vi "设备配置界面.vi"() -> ()   [LabVIEW 2016, in "环境动力监测库.lvlib"]
panel:
  in  "配置说明":bool
  in  "设置默认配置":bool
  in  "一键恢复默认设置":bool
  in  "add2":bool
  in  "串口连接":T1(ring)
  in  "设备列表":i32(listbox)=-1
  in  "add":bool
  in  "IO连接":T2(ring)
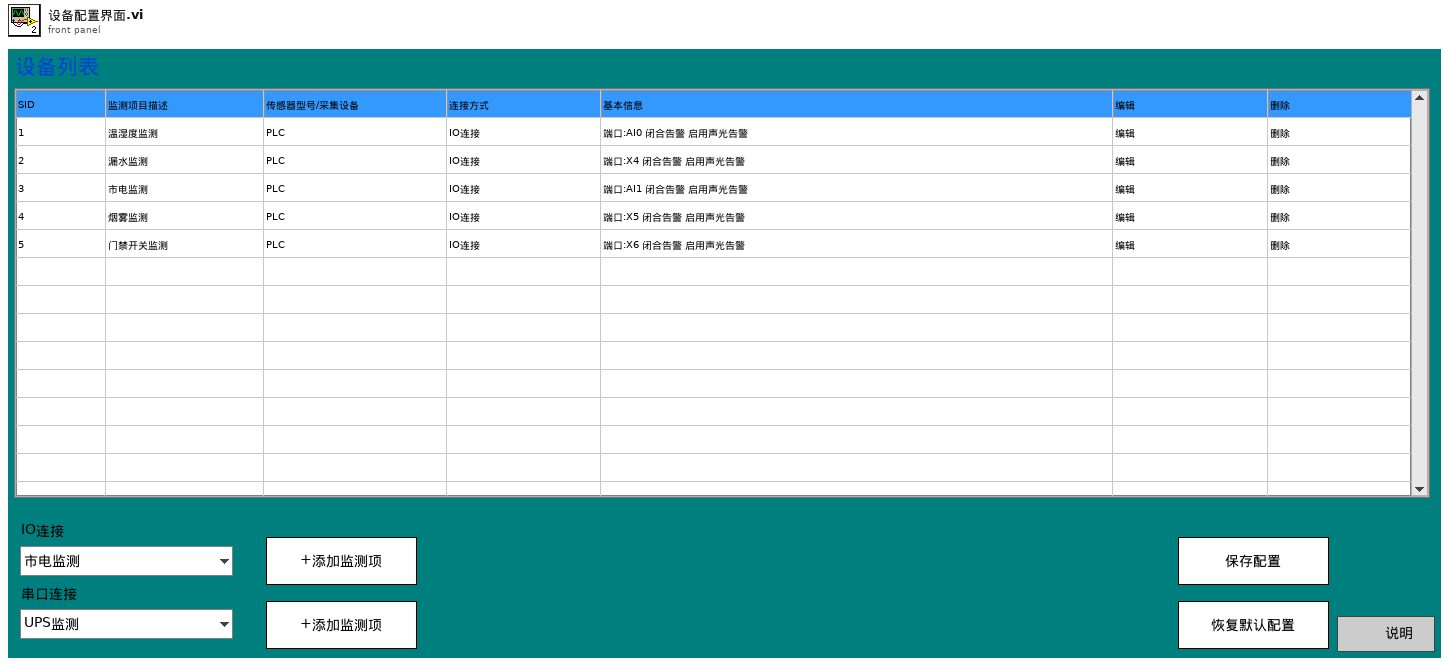
[diagram p1: front panel]
types:
  T1 = enum16{"UPS监测", "空调监测", "蓄电池监测", "GPS监测", "北斗监测", "智能门禁监测"}
  T2 = enum16{"市电监测", "用水量监测", "烟雾监测", "温湿度监测", "振动监测", "红外入侵监测", "漏水监测", "门禁开关监测", "视频监测", "冰箱监测", "排气扇监测", "废液监测"}
  T3 = cluster{"监测项描述:输出":string, "端口":enum16{"AI0", "AI1", "AI2", "AI3", "AI4", "DI0", "DI1", "DI2", "DI3", "DI4", "DI5", "DI6", "DI7", "DO0", "DO1", "DO2", "DO3", "DO4", "DO5", "DO6", "DO7", "X0", "X1", "X2", "X3", "X4", "X5", "X6", "X7", "X8", "X9", "X10", "X11", "X12", "X13", "X14", "X15", "X16", "X17", "X18", "X19", "X20", "X21", "X22", "X23", "Y0", "Y1", "Y2", "Y3", "Y4", "Y5", "Y6", "Y7", "Y8", "Y9", "Y10", "Y11", "Y12", "Y13", "Y14", "Y15", "Y16", "Y17", "Y18", "Y19", "Y20", "Y21", "Y22", "Y23", "Y24", "Y25", "Y26", "Y27", "Y28", "Y29", "Y30", "Y31", "Y32", "Y33", "Y34", "Y35", "Y36", "Y37", "Y38", "Y39"}, "告警方式":enum32{"禁用告警", "闭合告警", "断开告警"}, "传感器型号":enum16{"PLC", "ZLAN", "ART"}, "声光告警启用":bool}
  T4 = cluster{"监测项描述:输出":string, "连接方式":enum16{"串口", "TCP"}, "端口":string, "IP address:":string, "Port:":string, "站号":u64, "传感器型号":string, "波特率":u64, "data bits":u64, "停止位":u16, "奇偶校验":u16, "声光告警启用":bool}
  T5 = typedef "LVPoint32TypeDef.ctl" = cluster{"Horizontal":i32, "Vertical":i32}
  T6 = typedef "LVRowAndColumnTypeDef.ctl" = cluster{"Row":i32, "Column":i32}
  T7 = enum16{"Left Button", "Center Button", "Right Button", "Window Close"}
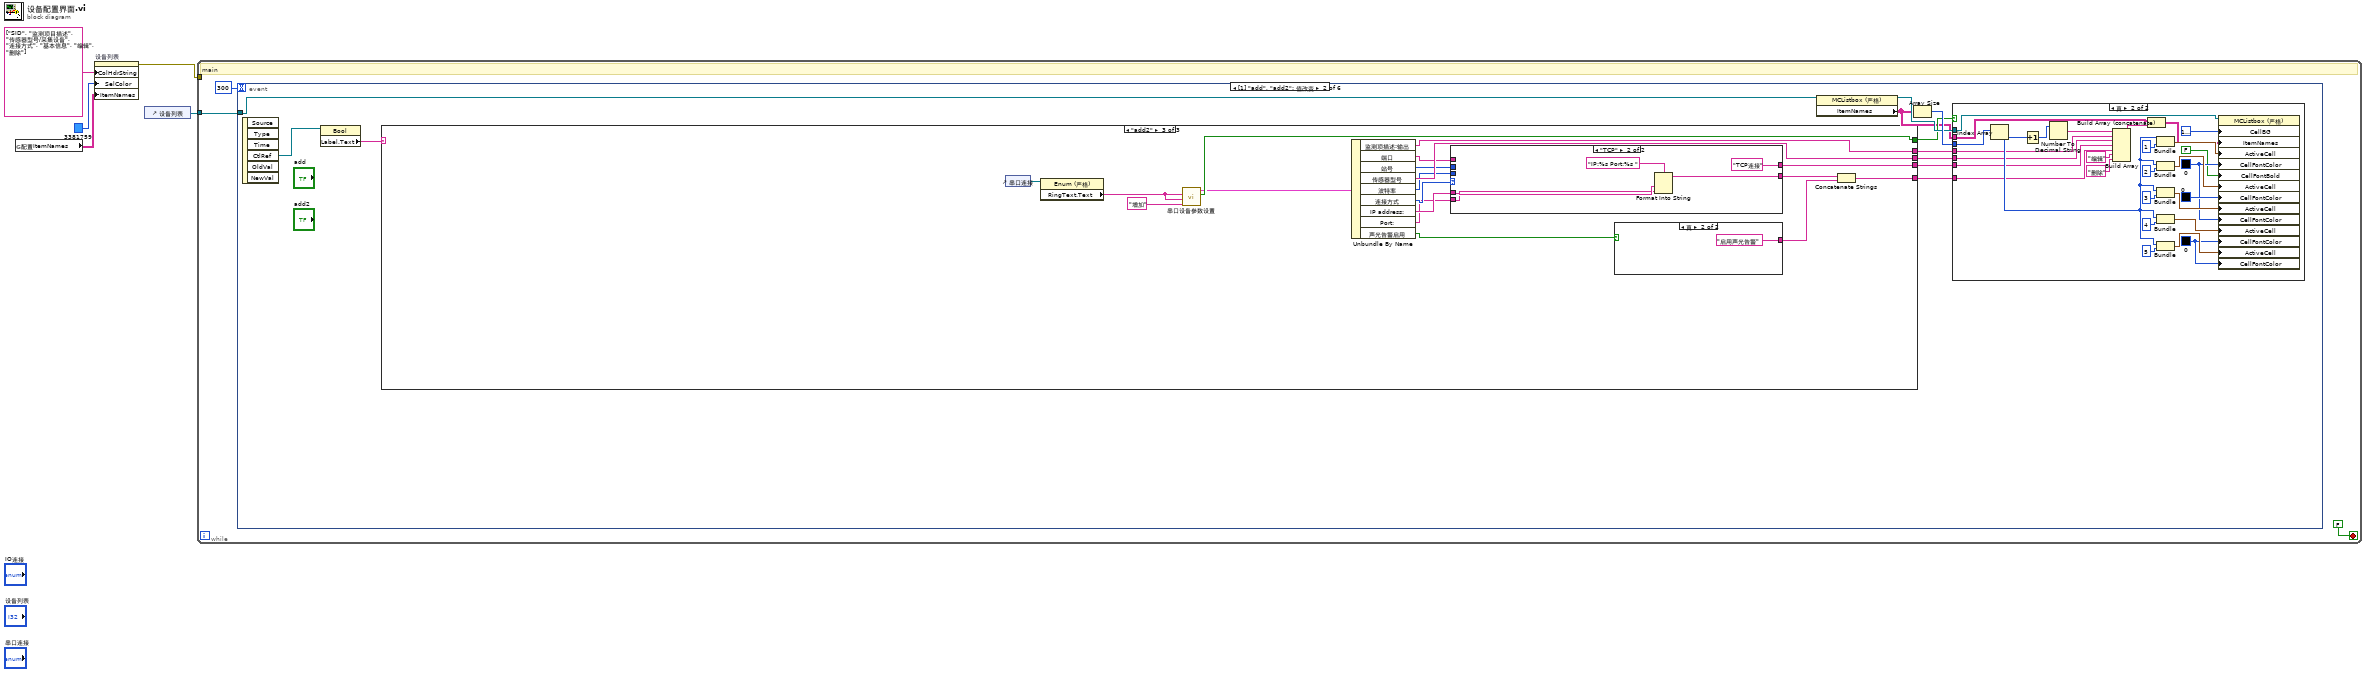
[diagram p0: block diagram]
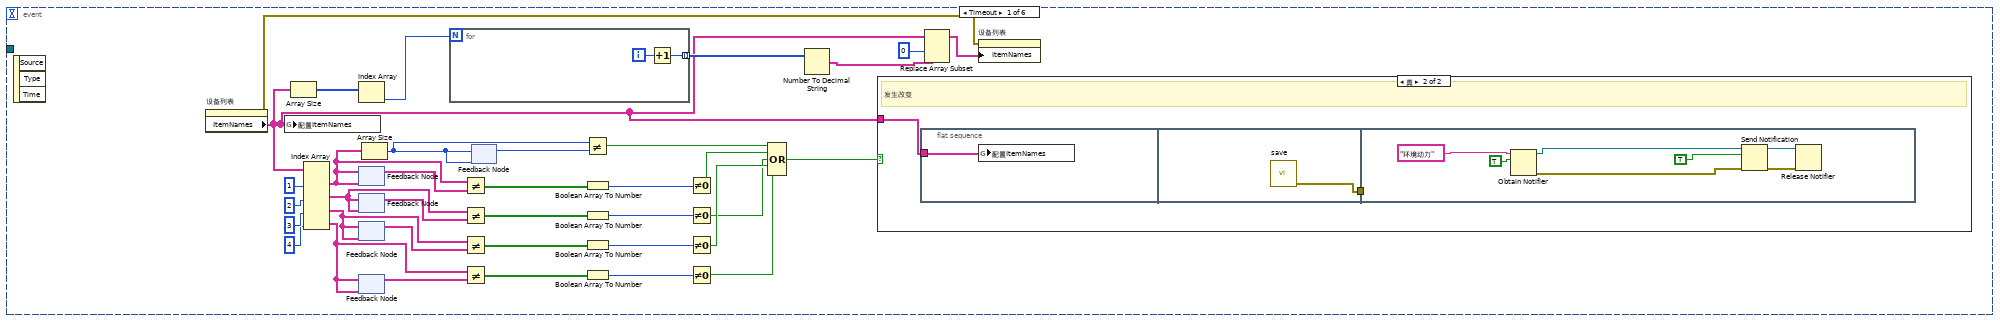
[diagram p2: hidden frame]
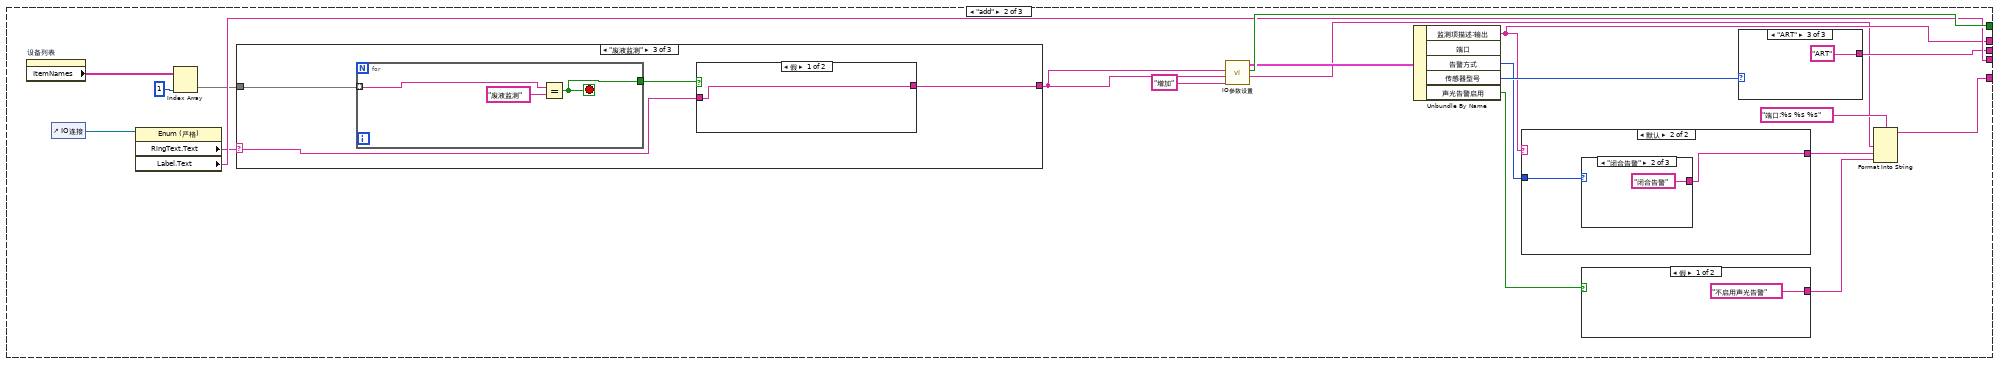
[diagram p5: hidden frame]
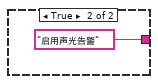
[diagram p6: hidden frame]
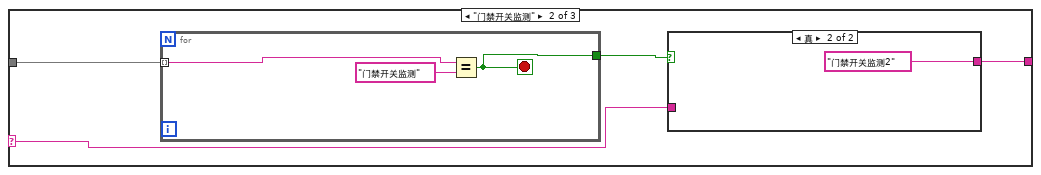
[diagram p8: hidden frame]
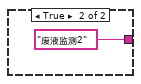
[diagram p10: hidden frame]
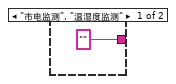
[diagram p11: hidden frame]
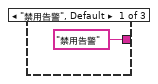
[diagram p12: hidden frame]
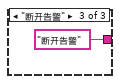
[diagram p13: hidden frame]
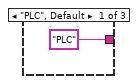
[diagram p14: hidden frame]
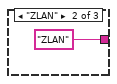
[diagram p15: hidden frame]
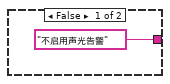
[diagram p16: hidden frame]
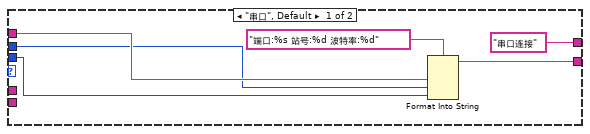
[diagram p17: hidden frame]
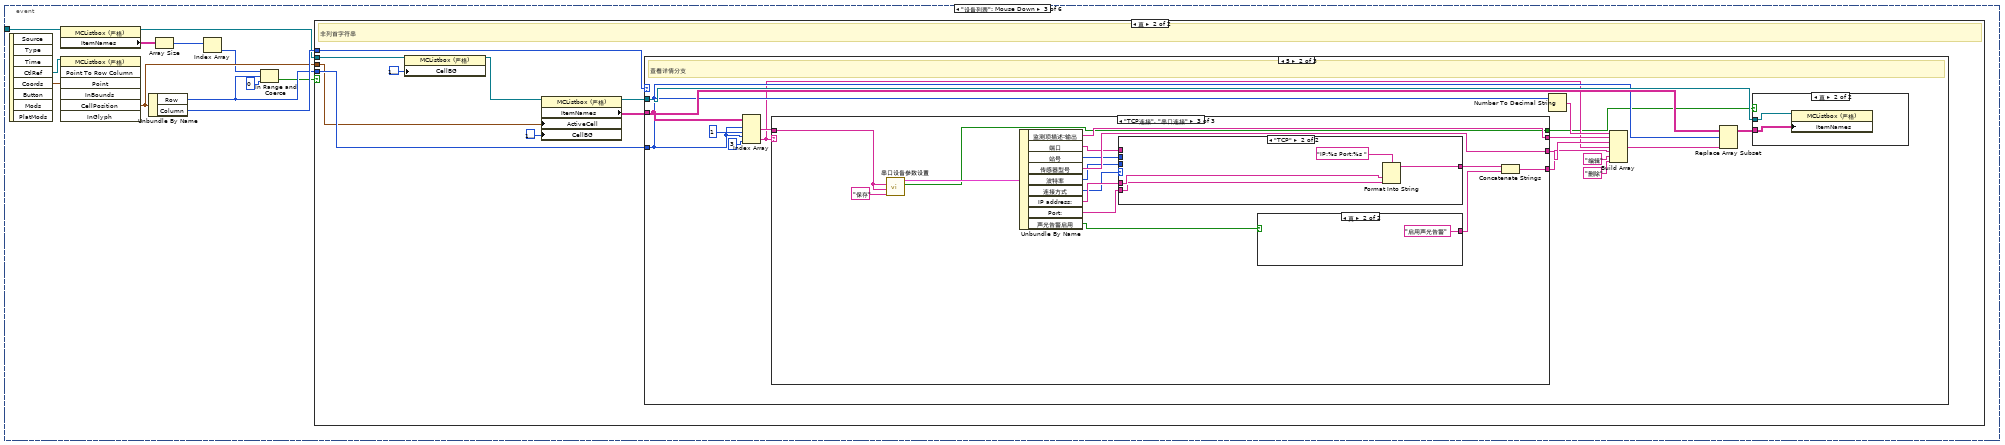
[diagram p19: hidden frame]
diagram:
  n1 = global read "断电保存全局变量.vi" "配置ItemNames"() -> (w1:string[][])
  n2 = property on="设备列表" class="MCListbox (严格)"("ColHdrString"=string[] ["SID", "监测项目描述", "传感器型号/采集设备", "连接方式", "基本信息", "编辑", "删除"] ("列首字符串[]"), "SelColor"=u32 3381759, "ItemNames"=w1) -> (error out=w4:errorcluster)  [unwired: 2 in, 1 out]
  n3 = control-ref of="设备列表"() -> (w5:refnum<vi>)
  n4 = while {
    tunnel: w5 -> [w7]
    tunnel: w4 -> [_]
    stop <- FALSE stop-if-true
    # "main"
    n5 = event shown="[1] \"add\", \"add2\": 值改变" {
      selector: _ -> [_ _ _ _ _ _]
      dyn-events: _ -> [_ _ _ _ _ _]
      timeout: 300 -> [_ _ _ _ _ _]
      tunnel: w7 -> [_ w68 w184 _ _ _]
      event Timeout {
        n6 = event-data() -> ()  [unwired: 1 in, 3 out]
        n7 = property on="设备列表" class="MCListbox (严格)"() -> (error out=w43:errorcluster, "ItemNames"=w9:string[][])  [unwired: 2 in, 1 out]
        n8 = global write "断电保存全局变量.vi" "配置ItemNames"(w9) -> ()
        n9 = Array Size(array=w9) -> (size(s)=w44:i32[])
        n10 = Index Array(array=w9, index (col) #1=1 ("禁用的索引 (列)"), index (col) #2=2 ("索引 (列)"), index (col) #3=3 ("索引 (列)"), index (col) #4=4 ("索引 (列)")) -> (element #1=w14:string[], element #2=w21:string[], element #3=w20:string[], element #4=w19:string[])  [unwired: 4 in]
        n11 = Index Array(array=w44) -> (element=w38:i32)  [unwired: 1 in]
        n12 = feedback-in #1(w14) -> ()
        n13 = feedback #1(w14) -> (w33:string[])
        n14 = feedback #2(w21) -> (w28:string[])
        n15 = feedback-in #2(w21) -> ()
        n16 = feedback #3(w20) -> (w27:string[])
        n17 = feedback-in #3(w20) -> ()
        n18 = feedback #4(w19) -> (w22:string[])
        n19 = feedback-in #4(w19) -> ()
        n20 = Array Size(array=w14) -> (size(s)=w12:i32)
        n21 = for {
          N: w38 -> [_]
          tunnel: [w56] -> w42 mode=indexing
          i -> [w57]
          n22 = Increment(x=w57) -> (x+1=w56:i32)
        }
        n23 = Not Equal?(x=w14, y=w33) -> (x != y?=w13:bool[])
        n24 = Not Equal?(x=w21, y=w28) -> (x != y?=w29:bool[])
        n25 = Not Equal?(x=w20, y=w27) -> (x != y?=w26:bool[])
        n26 = Not Equal?(x=w19, y=w22) -> (x != y?=w23:bool[])
        n27 = feedback #5(w12) -> (w11:i32)
        n28 = feedback-in #5(w12) -> ()
        n29 = Not Equal?(x=w12, y=w11) -> (x != y?=w10:bool)
        n30 = Boolean Array To Number(Boolean array=w13) -> (number=w32:u32)
        n31 = Boolean Array To Number(Boolean array=w29) -> (number=w30:u32)
        n32 = Boolean Array To Number(Boolean array=w26) -> (number=w25:u32)
        n33 = Boolean Array To Number(Boolean array=w23) -> (number=w24:u32)
        n34 = Not Equal To 0?(x=w32) -> (x != 0?=w31:bool)
        n35 = Not Equal To 0?(x=w30) -> (x != 0?=w16:bool)
        n36 = Not Equal To 0?(x=w25) -> (x != 0?=w17:bool)
        n37 = Not Equal To 0?(x=w24) -> (x != 0?=w18:bool)
        n38 = Compound Arithmetic op=OR ("复合运算")(w10, w31, w16, w17, w18) -> (w15:bool)
        n39 = Number To Decimal String(number=w42) -> (decimal integer string=w41:string[])  [unwired: 1 in]
        n40 = case shown="真" w15 {
          tunnel: w9 -> [_ w46]
          frame False {
          }
          frame True {
            # "发生改变"
            n41 = flat-sequence {
              tunnel: w46 -> [w47]
              tunnel: [w48] -> w45
              tunnel: w45 -> [_]
              frame #0 {
                n42 = global write "断电保存全局变量.vi" "配置ItemNames"(w47) -> ()
              }
              frame #1 {
                n43 = call "save.vi"() -> ("error out"=w48:errorcluster)  [unwired: 11 in]
              }
              frame #2 {
                n44 = Obtain Notifier(name (unnamed)="环境动力" ("名称（未命名）"), notification data type=TRUE) -> (notifier out=w51:refnum<notifier>, error out=w52:errorcluster)  [unwired: 2 in, 1 out]
                n45 = Send Notification(notification=TRUE ("通知"), notifier=w51, error in (no error)=w52) -> (notifier out=w54:refnum<notifier>, error out=w55:errorcluster)
                n46 = Release Notifier(notifier=w54, error in (no error)=w55) -> ()  [unwired: 1 in, 3 out]
              }
            }
          }
        }
        n47 = Replace Array Subset(array=w9, new element=w41, index (col)=0 ("禁用的索引 (列)")) -> (w39:string[][])  [unwired: 1 in]
        n48 = property on="设备列表" class="MCListbox (严格)"(error in=w43, "ItemNames"=w39) -> ()  [unwired: 1 in, 2 out]
      }
      event "add", "add2": Value Change {
        n49 = event-data() -> ("CtlRef"=w63:refnum<vi>)  [unwired: 1 in, 5 out]
        n50 = property class="Bool"(reference=w63) -> ("Label.Text"=w62:string)  [unwired: 1 in, 2 out]
        n51 = case shown="\"add2\"" w62 {
          tunnel: [_ w88 w135] -> w65
          tunnel: [_ w85 w119] -> w61
          tunnel: [_ w77 w131] -> w60
          tunnel: [_ w80 w130] -> w59
          tunnel: [_ w82 w120] -> w58
          frame "假", Default {
          }
          frame "add" {
            n52 = property on="设备列表" class="MCListbox (严格)"() -> ("ItemNames"=w71:string[][])  [unwired: 2 in, 2 out]
            n53 = control-ref of="IO连接"() -> (w86:refnum<vi>)
            n54 = property class="Enum (严格)"(reference=w86) -> ("RingText.Text"=w73:string, "Label.Text"=w85:string)  [unwired: 1 in, 2 out]
            n55 = Index Array(array=w71, index (col)=1 ("禁用的索引 (列)")) -> (element=w70:string[])  [unwired: 1 in]
            n56 = case shown="\"废液监测\"" w73 {
              selector: w73 -> [w91 w92 w101]
              tunnel: [w91 w95 w104] -> w76
              tunnel: w70 -> [_ w93 w102]
              frame "假", Default {
              }
              frame "门禁开关监测" {
                n57 = for {
                  tunnel: w93 -> [w100] mode=indexing
                  tunnel: [w98] -> w94
                  stop <- w98 stop-if-true
                  n58 = Equal?(x=w100, y="门禁开关监测") -> (x = y?=w98:bool)
                }
                n59 = case shown="真" w94 {
                  tunnel: w92 -> [w96 _]
                  tunnel: [w96 "门禁开关监测2" ("y")] -> w95
                  frame False {
                  }
                  frame True {
                  }
                }
              }
              frame "废液监测" {
                n60 = for {
                  tunnel: w102 -> [w109] mode=indexing
                  tunnel: [w107] -> w103
                  stop <- w107 stop-if-true
                  n61 = Equal?(x=w109, y="废液监测") -> (x = y?=w107:bool)
                }
                n62 = case shown="假" w103 {
                  tunnel: w101 -> [w105 _]
                  tunnel: [w105 "废液监测2" ("y")] -> w104
                  frame False {
                  }
                  frame True {
                  }
                }
              }
            }
            n63 = call "IO参数设置.vi"("布尔文本.文本"="增加", "section (optional)"=w76, "监测项描述"=w76) -> ("端口"=w69:string, "增加？"=w88:bool, "簇1输出"=w84:T3)  [unwired: 6 in]
            n64 = Unbundle By Name(w84) -> ("监测项描述:输出"=w77:string, "告警方式"=w79:enum32{"禁用告警", "闭合告警", "断开告警"}, "传感器型号"=w81:enum16{"PLC", "ZLAN", "ART"}, "声光告警启用"=w75:bool)  [unwired: 1 out]
            n65 = case shown="默认" w77 {
              tunnel: w79 -> [_ w112]
              tunnel: ["" w111] -> w78
              frame "市电监测", "温湿度监测" {
              }
              frame Default {
                n66 = case shown="\"闭合告警\"" w112 {
                  tunnel: ["禁用告警" "闭合告警" "断开告警"] -> w111
                  frame "禁用告警", Default {
                  }
                  frame "闭合告警" {
                  }
                  frame "断开告警" {
                  }
                }
              }
            }
            n67 = case shown="假" w75 {
              tunnel: ["不启用声光告警" "启用声光告警"] -> w74
              frame False {
              }
              frame True {
              }
            }
            n68 = case shown="\"ART\"" w81 {
              tunnel: ["PLC" "ZLAN" "ART"] -> w80
              frame "PLC", Default {
              }
              frame "ZLAN" {
              }
              frame "ART" {
              }
            }
            n69 = Format Into String(format string="端口:%s %s %s" ("格式字符串"), w69, w78, w74) -> (resulting string=w82:string)  [unwired: 2 in, 1 out]
          }
          frame "add2" {
            n70 = control-ref of="串口连接"() -> (w133:refnum<vi>)
            n71 = property class="Enum (严格)"(reference=w133) -> ("RingText.Text"=w134:string)  [unwired: 1 in, 2 out]
            n72 = call "串口设备参数设置.vi"("布尔文本.文本"="增加" ("section (optional)"), "section (optional)"=w134, "监测项描述"=w134) -> ("布尔"=w135:bool, "输出簇"=w132:T4)  [unwired: 7 in]
            n73 = Unbundle By Name(w132) -> ("监测项描述:输出"=w131:string, "端口"=w128:string, "站号"=w127:u64, "传感器型号"=w130:string, "波特率"=w126:u64, "连接方式"=w129:enum16{"串口", "TCP"}, "IP address:"=w125:string, "Port:"=w124:string, "声光告警启用"=w123:bool)
            n74 = case shown="\"TCP\"" w129 {
              tunnel: [w143 w146] -> w121
              tunnel: w128 -> [w142 _]
              tunnel: w127 -> [w141 _]
              tunnel: w126 -> [w140 _]
              tunnel: w125 -> [_ w148]
              tunnel: w124 -> [_ w147]
              tunnel: ["串口连接" "TCP连接"] -> w119
              frame "串口", Default {
                n75 = Format Into String(format string="端口:%s 站号:%d 波特率:%d" ("格式字符串"), w142, w141, w140) -> (resulting string=w143:string)  [unwired: 2 in, 1 out]
              }
              frame "TCP" {
                n76 = Format Into String(format string="IP:%s Port:%s " ("格式字符串"), w148, w147) -> (resulting string=w146:string)  [unwired: 2 in, 1 out]
              }
            }
            n77 = case shown="真" w123 {
              tunnel: ["不启用声光告警" ("格式字符串") "启用声光告警" ("格式字符串")] -> w122
              frame False {
              }
              frame True {
              }
            }
            n78 = Concatenate Strings(w121, w122) -> (w120:string)
          }
        }
        n79 = property class="MCListbox (严格)"(reference=w68) -> (reference out=w66:refnum<vi>, "ItemNames"=w64:string[][])  [unwired: 1 in, 1 out]
        n80 = Array Size(array=w64) -> (size(s)=w67:i32[])
        n81 = case shown="真" w65 {
          tunnel: w64 -> [_ w177]
          tunnel: w67 -> [_ w176]
          tunnel: w66 -> [_ w174]
          tunnel: w61 -> [_ w156]
          tunnel: w60 -> [_ w153]
          tunnel: w59 -> [_ w152]
          tunnel: w58 -> [_ w151]
          frame False {
          }
          frame True {
            w157 = u32 0 ("颜色盒")
            w164 = u32 0 ("颜色盒")
            n82 = Index Array(array=w176) -> (element=w159:i32)  [unwired: 1 in]
            n83 = Increment(x=w159) -> (x+1=w175:i32)
            n84 = Number To Decimal String(number=w175) -> (decimal integer string=w154:string)  [unwired: 1 in]
            n85 = Build Array(w154, w153, w152, w156, w151, "编辑" ("元素"), "删除" ("元素")) -> (w178:string[])
            n86 = Build Array (concatenate)(w177, w178) -> (w155:string[][])
            n87 = Bundle(w159, "Column"=1) -> (w165:cluster{i32, "Column":i32})  [unwired: 1 in]
            n88 = Bundle(w159, "Column"=2) -> (w171:cluster{i32, "Column":i32})  [unwired: 1 in]
            n89 = Bundle(w159, "Column"=3) -> (w168:cluster{i32, "Column":i32})  [unwired: 1 in]
            n90 = Bundle(w159, "Column"=4) -> (w166:cluster{i32, "Column":i32})  [unwired: 1 in]
            n91 = Bundle(w159, "Column"=5) -> (w158:cluster{i32, "Column":i32})  [unwired: 1 in]
            n92 = property class="MCListbox (严格)"(reference=w174, "CellBG"=u32 16777216 ("颜色盒"), "ItemNames"=w155, "ActiveCell"=w165, "CellFontColor"=w164, "CellFontBold"=FALSE ("活动单元格:单元格字体:斜体"), "ActiveCell"=w171, "CellFontColor"=u32 0 ("颜色盒"), "ActiveCell"=w168, "CellFontColor"=w164, "ActiveCell"=w166, "CellFontColor"=w157, "ActiveCell"=w158, "CellFontColor"=w157) -> ()  [unwired: 1 in, 2 out]
          }
        }
      }
      event "设备列表": Mouse Down {
        n93 = event-data() -> ("CtlRef"=w190:refnum<vi>, "Coords"=w188:T5)  [unwired: 1 in, 6 out]
        n94 = property class="MCListbox (严格)"(reference=w184) -> (reference out=w180:refnum<vi>, "ItemNames"=w183:string[][])  [unwired: 1 in, 1 out]
        n95 = invoke class="MCListbox (严格)" method="Point To Row Column"(reference=w190, "Point"=w188) -> ("CellPosition"=w187:T6)  [unwired: 5 in, 6 out]
        n96 = Unbundle By Name(w187) -> ("Row"=w186:i32, "Column"=w189:i32)
        n97 = Array Size(array=w183) -> (size(s)=w182:i32[])
        n98 = Index Array(array=w182) -> (element=w181:i32)  [unwired: 1 in]
        n99 = In Range and Coerce(upper limit=w181, x=w186, lower limit=0 ("下限")) -> (In Range?=w179:bool)  [unwired: 1 out]
        n100 = case shown="真" w179 {
          tunnel: w189 -> [_ w198]
          tunnel: w186 -> [_ w197]
          tunnel: w187 -> [_ w195]
          tunnel: w180 -> [_ w192]
          frame False {
          }
          frame True {
            # "非列首字符串"
            n101 = property class="MCListbox (严格)"(reference=w192, "CellBG"=u32 16777216) -> (reference out=w193:refnum<vi>)  [unwired: 1 in, 1 out]
            n102 = property class="MCListbox (严格)"(reference=w193, "ActiveCell"=w195, "CellBG"=u32 16777216) -> (reference out=w196:refnum<vi>, "ItemNames"=w199:string[][])  [unwired: 1 in, 1 out]
            n103 = case shown="5" w198 {
              tunnel: w199 -> [_ w211 w277]
              tunnel: w197 -> [_ w206 w275]
              tunnel: w196 -> [_ w212 w276]
              frame 0, Default {
              }
              frame 5 {
                # "查看详情分支"
                n104 = Index Array(array=w211, index (row) #1=w206, index (col) #1=1 ("禁用的索引 (列)"), index (row) #2=w206, index (col) #2=3 ("禁用的索引 (列)")) -> (element #1=w214:string, element #2=w201:string)
                n105 = case shown="\"TCP连接\", \"串口连接\"" w201 {
                  tunnel: w214 -> [_ w226 w253]
                  tunnel: [_ w222 w256] -> w204
                  tunnel: [_ w228 w244] -> w202
                  tunnel: [_ w224 w255] -> w203
                  tunnel: [_ w227 w254] -> w200
                  frame "假", Default {
                  }
                  frame "IO连接" {
                    n106 = call "IO参数设置.vi"("布尔文本.文本"="保存", "section (optional)"=w226, "监测项描述"=w226) -> ("端口"=w218:string, "增加？"=w227:bool, "簇1输出"=w229:T3)  [unwired: 6 in]
                    n107 = Unbundle By Name(w229) -> ("监测项描述:输出"=w222:string, "告警方式"=w223:enum32{"禁用告警", "闭合告警", "断开告警"}, "传感器型号"=w225:enum16{"PLC", "ZLAN", "ART"}, "声光告警启用"=w220:bool)  [unwired: 1 out]
                    n108 = case shown="\"市电监测\", \"温湿度监测\"" w222 {
                      tunnel: w223 -> [_ w236]
                      tunnel: ["" w235] -> w221
                      frame "市电监测", "温湿度监测" {
                      }
                      frame Default {
                        n109 = case shown="\"禁用告警\", 默认" w236 {
                          tunnel: ["禁用告警" "闭合告警" "断开告警"] -> w235
                          frame "禁用告警", Default {
                          }
                          frame "闭合告警" {
                          }
                          frame "断开告警" {
                          }
                        }
                      }
                    }
                    n110 = case shown="真" w220 {
                      tunnel: ["不启用声光告警" ("格式字符串") "启用声光告警" ("格式字符串")] -> w219
                      frame False {
                      }
                      frame True {
                      }
                    }
                    n111 = case shown="\"ART\"" w225 {
                      tunnel: ["PLC" "ZLAN" "ART"] -> w224
                      frame "PLC", Default {
                      }
                      frame "ZLAN" {
                      }
                      frame "ART" {
                      }
                    }
                    n112 = Format Into String(format string="端口:%s %s %s" ("格式字符串"), w218, w221, w219) -> (resulting string=w228:string)  [unwired: 2 in, 1 out]
                  }
                  frame "TCP连接", "串口连接" {
                    n113 = call "串口设备参数设置.vi"("布尔文本.文本"="保存", "section (optional)"=w253, "监测项描述"=w253) -> ("布尔"=w254:bool, "输出簇"=w257:T4)  [unwired: 7 in]
                    n114 = Unbundle By Name(w257) -> ("监测项描述:输出"=w256:string, "端口"=w249:string, "站号"=w248:u64, "传感器型号"=w255:string, "波特率"=w247:u64, "连接方式"=w250:enum16{"串口", "TCP"}, "IP address:"=w252:string, "Port:"=w251:string, "声光告警启用"=w246:bool)
                    n115 = case shown="\"TCP\"" w250 {
                      tunnel: [w264 w266] -> w245
                      tunnel: w249 -> [w263 _]
                      tunnel: w248 -> [w262 _]
                      tunnel: w247 -> [w261 _]
                      tunnel: w252 -> [_ w268]
                      tunnel: w251 -> [_ w267]
                      frame "串口", Default {
                        n116 = Format Into String(format string="端口:%s 站号:%d 波特率:%d" ("格式字符串"), w263, w262, w261) -> (resulting string=w264:string)  [unwired: 2 in, 1 out]
                      }
                      frame "TCP" {
                        n117 = Format Into String(format string="IP:%s Port:%s " ("格式字符串"), w268, w267) -> (resulting string=w266:string)  [unwired: 2 in, 1 out]
                      }
                    }
                    n118 = case shown="真" w246 {
                      tunnel: ["不启用声光告警" ("格式字符串") "启用声光告警" ("格式字符串")] -> w243
                      frame False {
                      }
                      frame True {
                      }
                    }
                    n119 = Concatenate Strings(w245, w243) -> (w244:string)
                  }
                }
                n120 = Number To Decimal String(number=w206) -> (decimal integer string=w205:string)  [unwired: 1 in]
                n121 = Build Array(w205, w204, w203, w201, w202, "编辑" ("元素"), "删除" ("元素")) -> (w207:string[])
                n122 = Replace Array Subset(array=w211, new element=w207, index (row)=w206) -> (w210:string[][])  [unwired: 1 in]
                n123 = case shown="真" w200 {
                  tunnel: w212 -> [_ w217]
                  tunnel: w210 -> [_ w216]
                  frame False {
                  }
                  frame True {
                    n124 = property class="MCListbox (严格)"(reference=w217, "ItemNames"=w216) -> ()  [unwired: 1 in, 2 out]
                  }
                }
              }
              frame 6 {
                # "删除"
                n125 = Index Array(array=w277, index (row)=w275, index (col)=1 ("禁用的索引 (列)")) -> (element=w271:string)
                n126 = Format Into String(format string="是否删除%s？" ("消息"), w271) -> (resulting string=w273:string)  [unwired: 2 in, 1 out]
                n127 = Two Button Dialog(message=w273) -> (T button?=w270:bool)  [unwired: 2 in]
                n128 = case shown="真" w270 {
                  tunnel: w276 -> [_ w282]
                  tunnel: w277 -> [_ w281]
                  tunnel: w275 -> [_ w280]
                  frame False {
                  }
                  frame True {
                    # "触发删除事件"
                    n129 = Delete From Array(array=w281, length=1 ("长度"), index (row)=w280) -> (array with subset deleted=w278:string[][])  [unwired: 1 in, 1 out]
                    n130 = property class="MCListbox (严格)"(reference=w282, "ItemNames"=w278) -> ()  [unwired: 1 in, 2 out]
                  }
                }
              }
            }
          }
        }
      }
      event "一键恢复默认设置": Value Change {
        n131 = event-data() -> ()  [unwired: 1 in, 6 out]
        n132 = call <vilib>:"Three Button Dialog.vi"("Center Button Text (\"No\")"="配置文件" ("Center Button Text (\"No\")"), "Left Button Text (\"Yes\")"="本机" ("Left Button Text (\"Yes\")"), "message"="请选择是否恢复默认？") -> ("Which Button?"=w284:T7)  [unwired: 8 in]
        n133 = case shown="\"Left Button\", 默认" w284 {
          frame "Left Button", Default {
            n134 = call "开机添加默认配置文件.vi"("恢复默认方式"=enum16{"无配置开机恢复", "手动恢复"}."手动恢复") -> ("error out"=w287:errorcluster)  [unwired: 10 in]
            n135 = case shown="无错误" w287 {
              frame No Error {
                n136 = One Button Dialog(message="配置成功！" ("消息")) -> (true=w289:bool)  [unwired: 1 in]
                n137 = case shown="真" w289 {
                  frame False {
                  }
                  frame True {
                    n138 = call "load.vi"() -> ("error out"=w291:errorcluster)  [unwired: 11 in]
                    n139 = flat-sequence {
                      tunnel: w291 -> [w292]
                      tunnel: [w292] -> _
                      frame #0 {
                        n140 = case shown="无错误" w292 {
                          frame No Error {
                            n141 = global read "断电保存全局变量.vi" "配置ItemNames"() -> (w294:string[][])
                            n142 = control-ref of="设备列表"() -> (w293:refnum<vi>)
                            n143 = property on="属性节点" class="MCListbox (严格)"(reference=w293, "ColHdrString"=string[] ["SID", "监测项目描述", "传感器型号/采集设备", "连接方式", "基本信息", "编辑", "删除"] ("列首字符串[]"), "SelColor"=u32 3381759, "ItemNames"=w294) -> ()  [unwired: 1 in, 2 out]
                          }
                          frame Error {
                          }
                        }
                      }
                    }
                  }
                }
              }
              frame Error {
                n144 = One Button Dialog(message="配置失败！" ("消息")) -> ()  [unwired: 1 in, 1 out]
              }
            }
          }
          frame "Center Button" {
            n145 = vi-ref "环境动力监测库.lvlib:断电保存全局变量.vi"() -> (w302:refnum<vi>)
            n146 = call "load config.vi"("TABLE"="power_environment_monitoring_default", "VI引用句柄"=w302) -> ("error out"=w299:errorcluster)  [unwired: 9 in]
            n147 = vi-ref "环境动力监测库.lvlib:断电保存全局变量.vi"() -> (w303:refnum<vi>)
            n148 = call "save config.vi"("error in (no error)"=w299, "TABLE"="power_environment_monitoring", "VI引用句柄"=w303) -> ("error out"=w298:errorcluster)  [unwired: 8 in]
            n149 = case shown="无错误" w298 {
              frame No Error {
                n150 = One Button Dialog(message="配置成功！" ("消息")) -> (true=w304:bool)  [unwired: 1 in]
                n151 = case shown="真" w304 {
                  frame False {
                  }
                  frame True {
                    n152 = call "load.vi"() -> ("error out"=w306:errorcluster)  [unwired: 11 in]
                    n153 = flat-sequence {
                      tunnel: w306 -> [w307]
                      tunnel: [w307] -> _
                      frame #0 {
                        n154 = case shown="无错误" w307 {
                          frame No Error {
                            n155 = global read "断电保存全局变量.vi" "配置ItemNames"() -> (w309:string[][])
                            n156 = control-ref of="设备列表"() -> (w308:refnum<vi>)
                            n157 = property on="属性节点" class="MCListbox (严格)"(reference=w308, "ColHdrString"=string[] ["SID", "监测项目描述", "传感器型号/采集设备", "连接方式", "基本信息", "编辑", "删除"] ("列首字符串[]"), "SelColor"=u32 3381759, "ItemNames"=w309) -> ()  [unwired: 1 in, 2 out]
                          }
                          frame Error {
                          }
                        }
                      }
                    }
                  }
                }
              }
              frame Error {
              }
            }
          }
          frame "Right Button" {
          }
          frame "Window Close" {
          }
        }
      }
      event "设置默认配置": Value Change {
        n158 = event-data() -> ()  [unwired: 1 in, 6 out]
        n159 = Two Button Dialog(message="确认将当前配置设置为默认配置？" ("消息")) -> (T button?=w312:bool)  [unwired: 2 in]
        n160 = case shown="真" w312 {
          frame False {
          }
          frame True {
            n161 = vi-ref "环境动力监测库.lvlib:断电保存全局变量.vi"() -> (w316:refnum<vi>)
            n162 = call "save config.vi"("TABLE"="power_environment_monitoring_default", "VI引用句柄"=w316) -> ("error out"=w314:errorcluster)  [unwired: 9 in]
            n163 = case shown="无错误" w314 {
              frame No Error {
                n164 = One Button Dialog(message="配置成功！" ("消息")) -> ()  [unwired: 1 in, 1 out]
              }
              frame Error {
                n165 = One Button Dialog(message="配置失败！" ("消息")) -> ()  [unwired: 1 in, 1 out]
              }
            }
          }
        }
      }
      event "配置说明": Value Change {
        n166 = event-data() -> ()  [unwired: 1 in, 6 out]
        n167 = vi-ref "环境动力监测库.lvlib:配置说明.vi"() -> (w319:refnum<vi>)
        n168 = property class="VI"(reference=w319) -> ("Name"=w320:string)  [unwired: 1 in, 2 out]
        n169 = Open VI Reference(type specifier VI Refnum (for type only)=refnum<vi> refnum, vi path=w320, options=128 ("选项")) -> (vi reference=w322:refnum<vi>, error out=w324:errorcluster)  [unwired: 3 in]
        n170 = call-by-ref "开始异步调用"(reference=w322, error in=w324) -> (reference out=w326:refnum<vi>, error out=w325:errorcluster)  [unwired: 11 in, 1 out]
        n171 = Close Reference(reference=w326, error in (no error)=w325) -> ()  [unwired: 1 out]
      }
    }
  }
